vi "TestPowerMeasure_WithSub.vi"() -> (0 "error out":errorcluster)   [LabVIEW 2012]
uses:
  TypeDefs/OphirRef.ctl
panel:
  out "OphirRef Out":T1
  out "mean":dbl format="%.6g"
  out "median":dbl format="%.6g"
  in  "error in (no error)":errorcluster
  in  "Measure":bool
  in  "Stop":bool
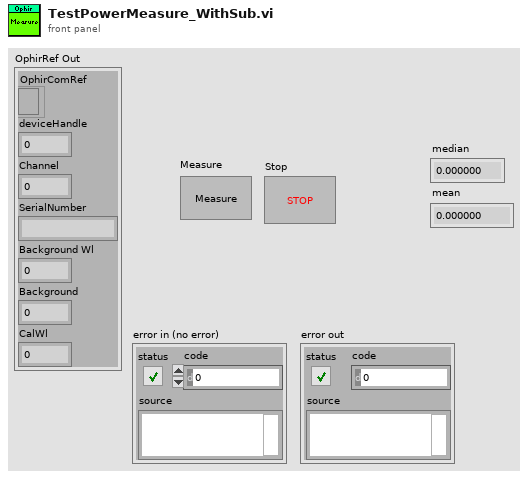
[diagram p1: front panel]
types:
  T1 = typedef "OphirRef.ctl" = cluster{"OphirComRef":refnum<k7>, "deviceHandle":i32, "Channel":i32, "SerialNumber":string, "Background Wl":dbl, "Background":dbl, "CalWl":dbl}
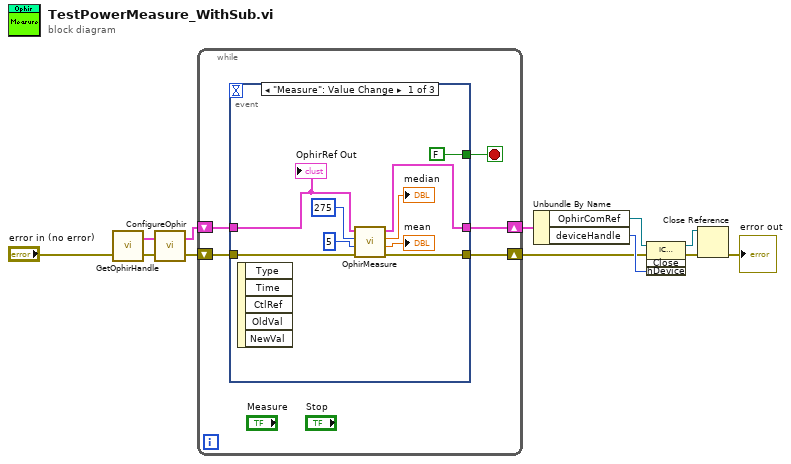
[diagram p0: block diagram]
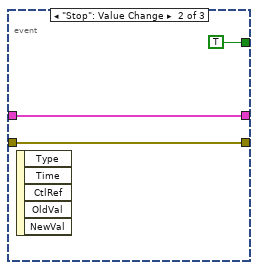
[diagram p2: hidden frame]
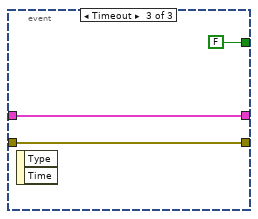
[diagram p3: hidden frame]
diagram:
  n1 = call "GetOphirHandle.vi"("error in (no error)"="error in (no error)") -> ("error out"=w8:errorcluster, "OphirRef Out"=w11:T1)  [unwired: 1 in]
  n2 = call "ConfigureOphir.vi"("error in (no error)"=w8, "OphirRef In"=w11) -> ("error out"=w9:errorcluster, "OphirRef Out"=w10:T1)
  n3 = while {
    shift-right: [w16] -> w4
    shift-left: w9 -> [w17]
    shift-right: [w13] -> w7
    shift-left: w10 -> [w14]
    stop <- w15 stop-if-true
    n4 = event shown="[0] \"Measure\": Value Change" {
      selector: _ -> [_ _ _]
      dyn-events: _ -> [_ _ _]
      timeout: _ -> [_ _ _]
      tunnel: w17 -> [w22 w28 w31]
      tunnel: [w21 w28 w31] -> w16
      tunnel: [FALSE ("Stop") TRUE ("Stop") FALSE ("Stop")] -> w15
      tunnel: w14 -> [w25 w27 w30]
      tunnel: [w18 w27 w30] -> w13
      event "Measure": Value Change {
        n5 = event-data() -> ()  [unwired: 1 in, 5 out]
        n6 = call "OphirMeasure.vi"("error in (no error)"=w22, "Samples"=5, "wavelength"=275, "OphirRef In"=w25) -> ("error out"=w21:errorcluster, "mean"=→"mean":dbl, "median"=→"median":dbl, "OphirRef Out"=w18:T1)
        "OphirRef Out" <- w25
      }
      event "Stop": Value Change {
        n7 = event-data() -> ()  [unwired: 1 in, 5 out]
      }
      event Timeout {
        n8 = event-data() -> ()  [unwired: 1 in, 2 out]
      }
    }
  }
  n9 = Unbundle By Name(w7) -> ("OphirComRef"=w6:refnum<k7>, "deviceHandle"=w5:i32)
  n10 = invoke class="ICoLMMeasurement2" method="Close"(reference=w6, error in=w4, "hDevice"=w5) -> (reference out=w3:refnum<k7>, error out=w2:errorcluster)  [unwired: 1 in, 2 out]
  n11 = Close Reference(reference=w3, error in (no error)=w2) -> (error out=→"error out":errorcluster)
